vi "HSPA_QAM_Tx.vi"() -> ()   [LabVIEW 2025]
uses:
  <vilib>/sound2/lvsound2.llb/Sound Data Format.ctl
  <vilib>/addons/Modulation/Analog/support/mod_Set Error Source.vi
  <vilib>/sound2/lvsound2.llb/Sound File Info (path).vi
  <vilib>/addons/Modulation/Digital/General/MT Generate QAM System Parameters(M).vi
  <vilib>/addons/Modulation/Digital/Support/Common/Validators/mod_Generate Filter Coefficients Validate.vi
  <vilib>/addons/Modulation/Digital/General/subVIs/mod_Generate Filter Coefficients.vi
  <instrlib>/niUSRP/niUSRP Write Tx Data (CDB).vi
  <vilib>/addons/Modulation/niDMT.lvlib
panel:
  out "Constellation Graph 2":T1(graph)
  in  "filter parameter":dbl=0.5 format="%.2f"
  out "constellation graph":T2(array[cluster]) {"oversampled data" format="%.2f"; "constellation" format="%.2f"}
  in  "samples per symbol (16)":i32=16
  out "data":waveform(dbl)[](array[waveform])
  out "sound format":T3={"sample rate (S/s)"=22050.0, "number of channels"=2, "bits per sample"=16}
  in  "matched samples per symbol (16)":i32=16
  in  "Path input":path
  in  "pulse shaping samples per symbol (16)":i32=16
  in  "pulse shaping filter (none)":T4(ring)
  out "error out":errorcluster
  in  "reset? (T)":bool=TRUE
  in  "active antenna":string
  in  "gain":dbl format="%#_6f"
  in  "carrier frequency":dbl=100000.0 format="%#_6p"
  in  "IQ rate":dbl=100000.0 format="%#_6p"
  in  "error in (no error)":errorcluster
  in  "USRP IP Address":refnum<k15>
  in  "stop":bool
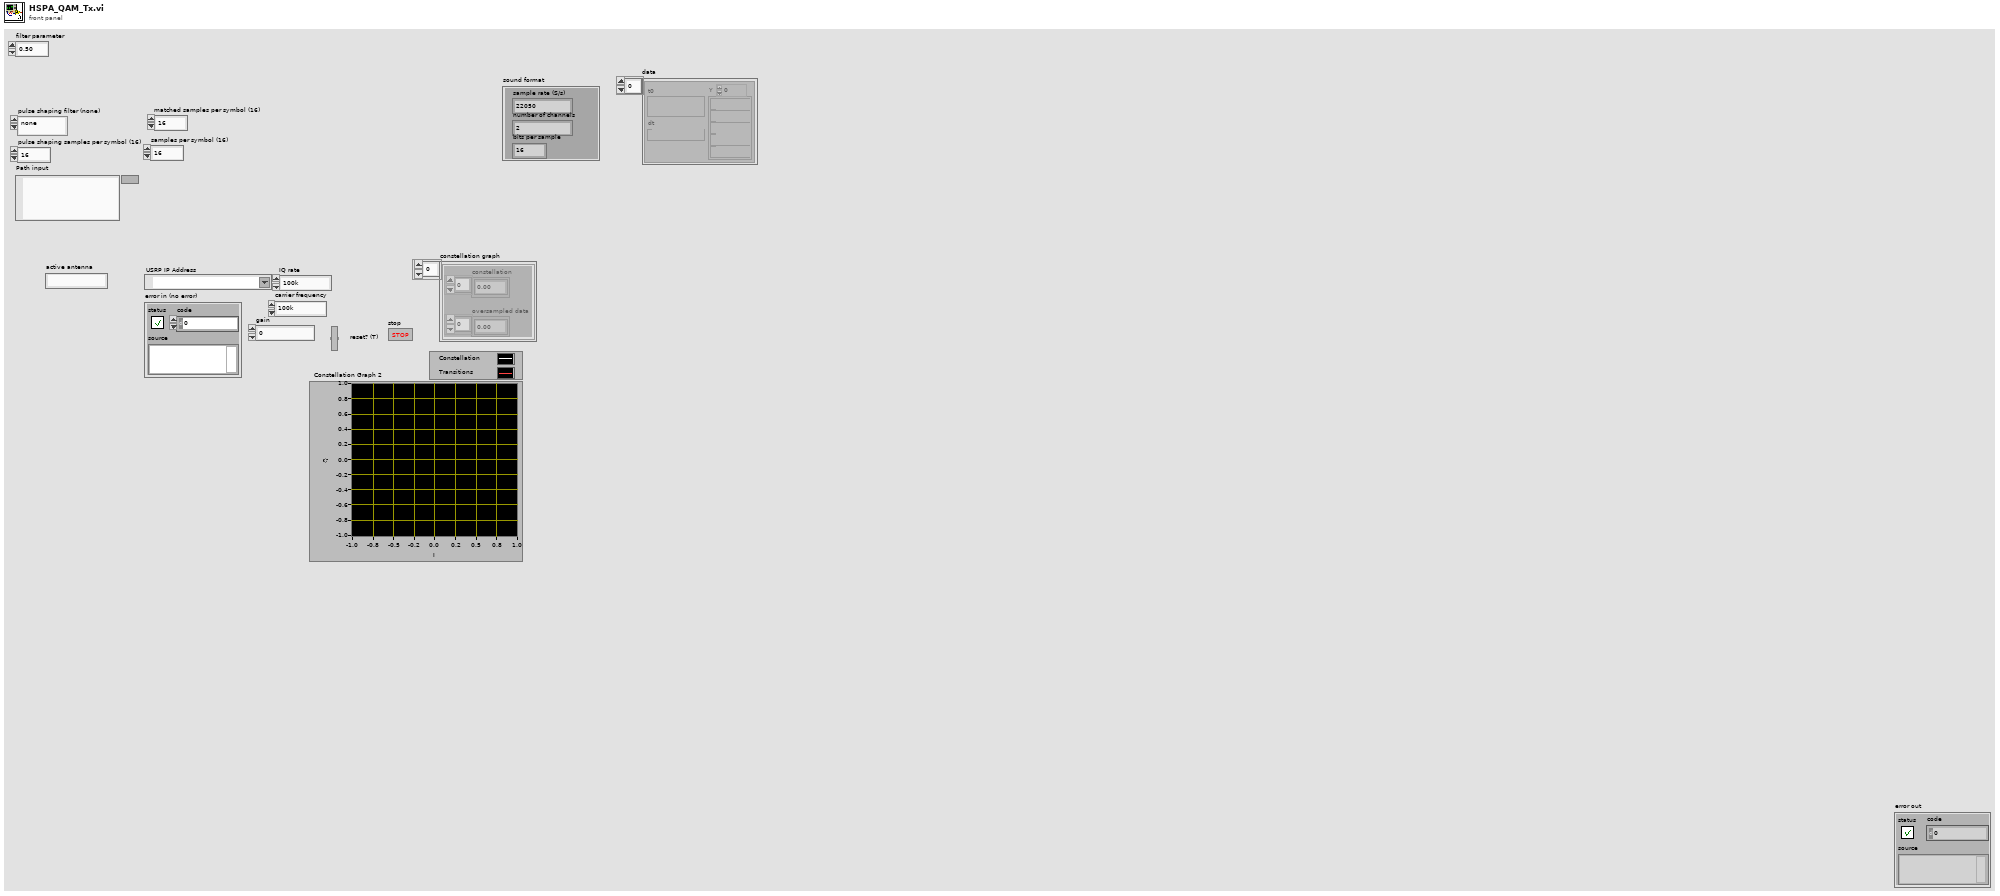
[diagram p1: front panel]
types:
  T1 = cluster{"Decimated Array":dbl[], "Decimated Array":dbl[]}[]
  T2 = cluster{"constellation":dbl[], "oversampled data":dbl[]}[]
  T3 = typedef "Sound Data Format.ctl" = cluster{"sample rate (S/s)":dbl, "number of channels":i32, "bits per sample":i32}
  T4 = enum16{"none", "Raised Cosine", "Root Raised Cos", "Gaussian"}
  T5 = enum16{"FSK", "PSK", "QAM", "MSK", "PAM", "ASK", "CPM"}
  T6 = cluster{"samples per symbol (16)":i32, "symbol map":cdb[]}
  T7 = typedef "niAMT.lvlib/Complex Data Waveform.ctl" = cluster{"t0":dbl, "dt":dbl, "Y":cdb[]}
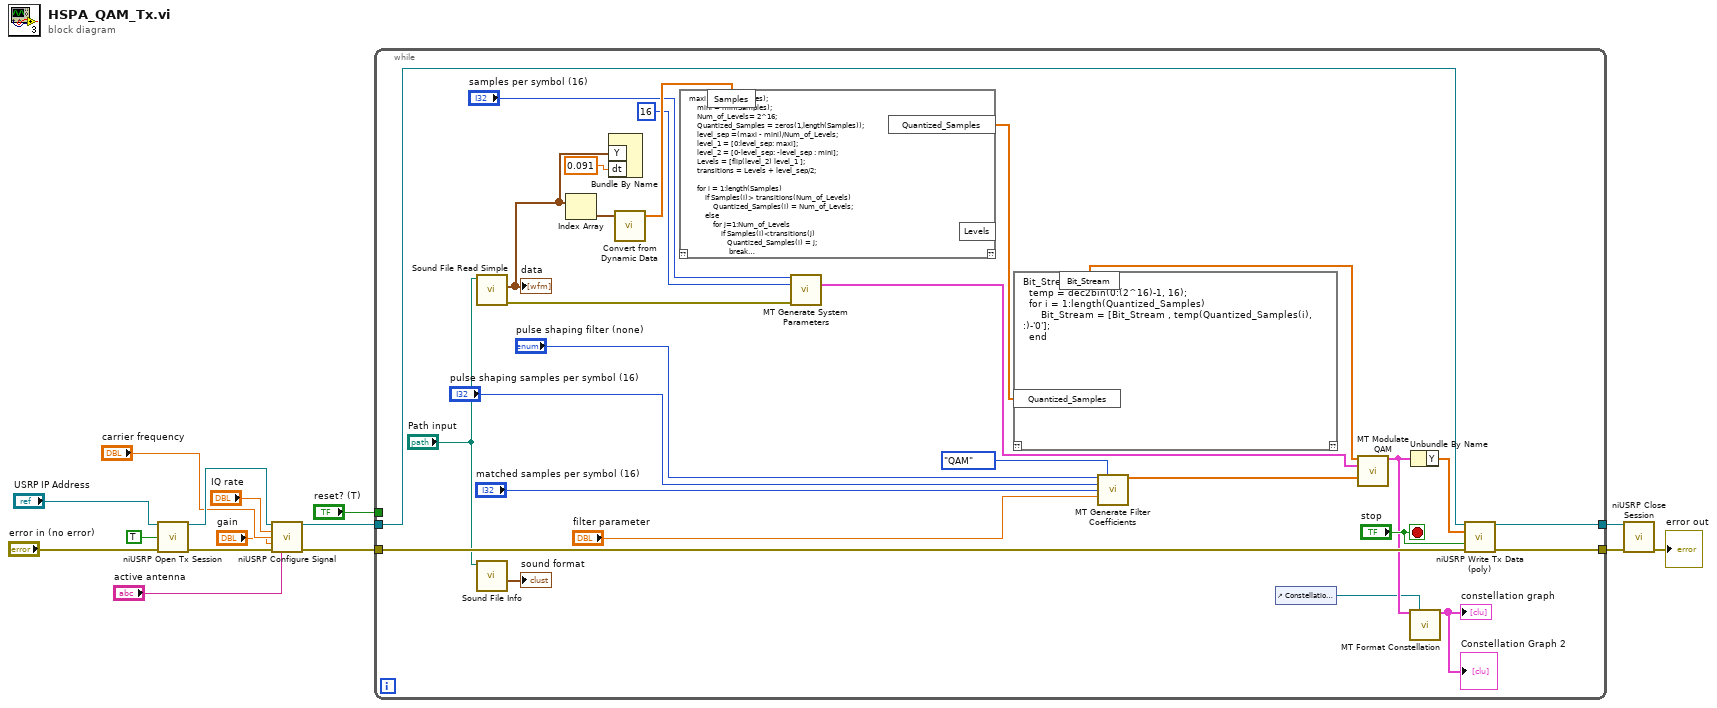
[diagram p0: block diagram]
diagram:
  n1 = call <instrlib>:"niUSRP Open Tx Session.vi"("device names"="USRP IP Address", "reset"=TRUE, "error in (no error)"="error in (no error)") -> ("session handle out"=w15:refnum<k15>, "error out"=w14:errorcluster)  [unwired: 11 in]
  n2 = call <instrlib>:"niUSRP Configure Signal.vi"("session handle"=w15, "IQ rate"="IQ rate", "carrier frequency"="carrier frequency", "gain"="gain", "error in (no error)"=w14, "active antenna"="active antenna") -> ("session handle out"=w3:refnum<k15>, "error out"=w7:errorcluster)  [unwired: 5 in, 3 out]
  n3 = while {
    tunnel: [w42] -> w4
    tunnel: [w41] -> w5
    tunnel: w7 -> [w38]
    tunnel: "reset? (T)" -> [_]
    tunnel: w3 -> [w39]
    stop <- "stop" stop-if-true
    n4 = call <vilib>:"Sound File Read Simple.vi"("path"="Path input") -> ("error out"=w26:errorcluster, "data"=w17:waveform(dbl)[])  [unwired: 7 in, 2 out]
    "data" <- w17
    n5 = call-poly <vilib>:"Sound File Info.vi"("path"="Path input") -> ("sound format"=→"sound format":T3)  [unwired: 7 in, 3 out]
    n6 = Index Array(array=w17) -> (element=w16:waveform(dbl))  [unwired: 1 in]
    n7 = Bundle By Name("Y"=w17, "dt"=0.091) -> ()  [unwired: 1 in, 1 out]
    n8 = call "Convert from Dynamic Data"("Dynamic Data Type"=w16) -> ("Array"=w30:dbl[])  [unwired: 3 in]
    n9 = script code="maxi = max(Samples);\n    mini = min(Samples);\n    Num_of_Levels= 2^16;\n    Quantized_Samples = zeros(1,length(Samples));\n    level_sep =(maxi - mini)/Num_of_Levels; \n    level_1 = [0:level_sep: maxi];\n    level_2 = [0-level_sep: -level_sep : mini];\n    Levels = [flip(level_2) level_1 ];\n    transitions = Levels + level_sep/2;\n    \n    for i = 1:length(Samples)\n        if Samples(i)> transitions(Num_of_Levels)\n            Quantized_Samples(i) = Num_of_Levels;\n        else\n            for j=1:Num_of_Levels\n                if Samples(i)<transitions(j)\n                   Quantized_Samples(i) = j;\n                    break\n                end\n            end\n        end\n    end"("Samples"=w30) -> ("Quantized_Samples"=w31:dbl[])  [unwired: 1 in, 2 out]
    n10 = call-poly <vilib>:"MT Generate System Parameters.vi"("samples per symbol (16)"="samples per symbol (16)", "M-QAM (16)"=16, "error in (no error)"=w26) -> ("QAM system parameters"=w25:T6)  [unwired: 10 in, 2 out]
    n11 = script code="Bit_Stream = [];\n  temp = dec2bin(0:(2^16)-1, 16);  \n  for i = 1:length(Quantized_Samples)\n      Bit_Stream = [Bit_Stream , temp(Quantized_Samples(i), :)-'0'];\n  end"("Quantized_Samples"=w31) -> ("Bit_Stream"=w24:dbl[])  [unwired: 1 in, 1 out]
    n12 = call <vilib>:"MT Generate Filter Coefficients.vi"("pulse shaping filter (none)"="pulse shaping filter (none)", "modulation type"=T5."QAM", "pulse shaping samples per symbol (16)"="pulse shaping samples per symbol (16)", "matched samples per symbol (16)"="matched samples per symbol (16)", "filter parameter"="filter parameter") -> ("pulse shaping filter coefficients"=w27:dbl[])  [unwired: 8 in, 2 out]
    n13 = control-ref of="Constellation Graph 2"() -> (w18:refnum<vi>)
    n14 = call <vilib>:"MT Modulate QAM.vi"("input bit stream"=w24, "QAM system parameters"=w25, "pulse shaping filter coefficients"=w27) -> ("output complex waveform"=w21:T7)  [unwired: 10 in, 2 out]
    n15 = call <vilib>:"MT Format Constellation.vi"("waveform"=w21, "constellation reference"=w18) -> ("constellation graph"=→"constellation graph" →"Constellation Graph 2":T2)  [unwired: 3 in, 10 out]
    n16 = Unbundle By Name(w21) -> ("Y"=w29:cdb[])
    n17 = call-poly <instrlib>:"niUSRP Write Tx Data (poly).vi"("session handle"=w39, "data"=w29, "end of data?"="stop", "error in (no error)"=w38) -> ("session handle out"=w41:refnum<k15>, "error out"=w42:errorcluster)  [unwired: 10 in]
  }
  n18 = call <instrlib>:"niUSRP Close Session.vi"("session handle"=w5, "error in (no error)"=w4) -> ("error out"=→"error out":errorcluster)  [unwired: 13 in]
